vi "数组至表格.vi"(10 "数组":sgl[][](array[numeric])) -> (2 "表格控件":string[][](table))   [LabVIEW 2010]
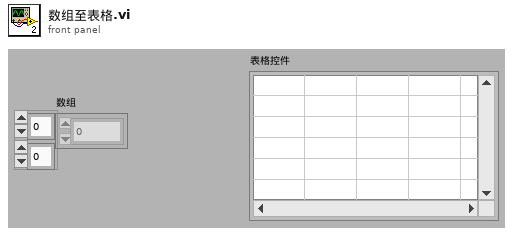
[diagram p1: front panel]
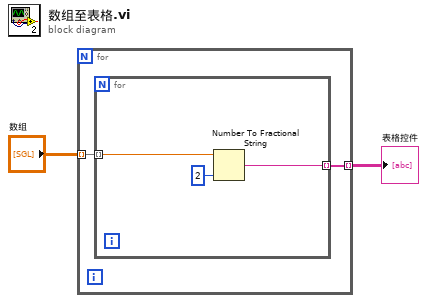
[diagram p0: block diagram]
diagram:
  n1 = for {
    tunnel: "数组" -> [w4] mode=indexing
    tunnel: [w3] -> w1 mode=indexing
    n2 = for {
      tunnel: w4 -> [w5] mode=indexing
      tunnel: [w6] -> w3 mode=indexing
      n3 = Number To Fractional String(number=w5, precision (6)=i16 2 ("精度(6)")) -> (F-format string=w6:string)  [unwired: 2 in]
    }
  }
  "表格控件" <- w1
